vi "pack.vi"(8 "error in (no error)":errorcluster, 11 "Bottle in":refnum<class "Bottle.lvclass">) -> (0 "error out":errorcluster, 2 "Packing":string, 3 "Bottle out":refnum<class "Bottle.lvclass">)   [LabVIEW 2018, in "Bottle.lvclass"]
uses:
  Bottle.lvclass
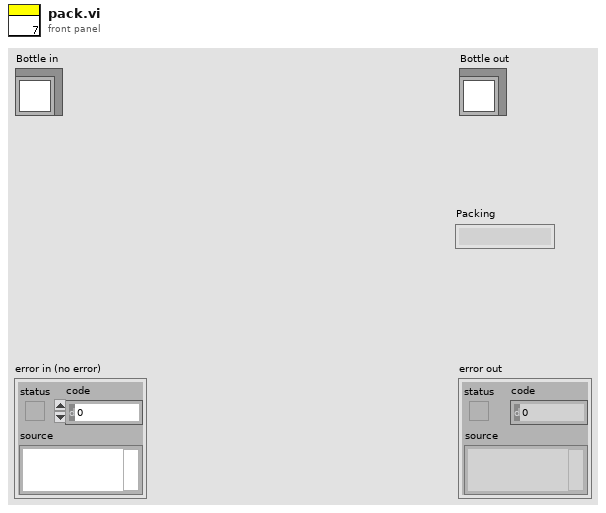
[diagram p1: front panel]
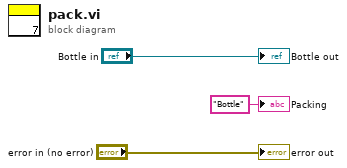
[diagram p0: block diagram]
diagram:
  "error out" <- "error in (no error)"
  "Bottle out" <- "Bottle in"
  "Packing" <- "Bottle" ("Packing")
